vi "MCLB_AssertDisabledItems_Tests.vi"(11 "error in":errorcluster) -> (15 "error out":errorcluster)   [LabVIEW 2016, in "DronaTest.lvlib"]
uses:
  DronaTest.lvlib
  APIs/Stimulus/ControlValue/SetValueAuto.vi
  APIs/Assert/AssertControlValue/Controls/MC Listbox/AssertDisabledItems.vi
  <vilib>/addons/_JKI Toolkits/Caraya/classes/Assert/Assert Error.vi
  <vilib>/addons/_JKI Toolkits/Caraya/classes/Assert/Assert Equal Value_Variant.vi
  <vilib>/addons/_JKI Toolkits/Caraya/classes/Test/Test.lvclass
  Drona.lvlib
  <vilib>/SLL Toolkit/SLL Debug/SLL Debug.lvlib
  <vilib>/addons/_JKI Toolkits/Caraya/classes/Assert/Assert.lvclass
  APIs/Stimulus/ControlValue/ControlValue.lvlib
  APIs/Assert/AssertControlValue/Controls/MC Listbox/AssertMCListbox.lvlib
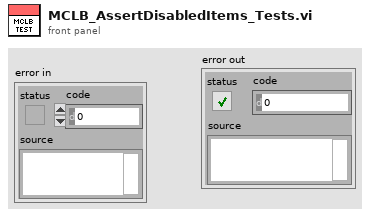
[diagram p1: front panel]
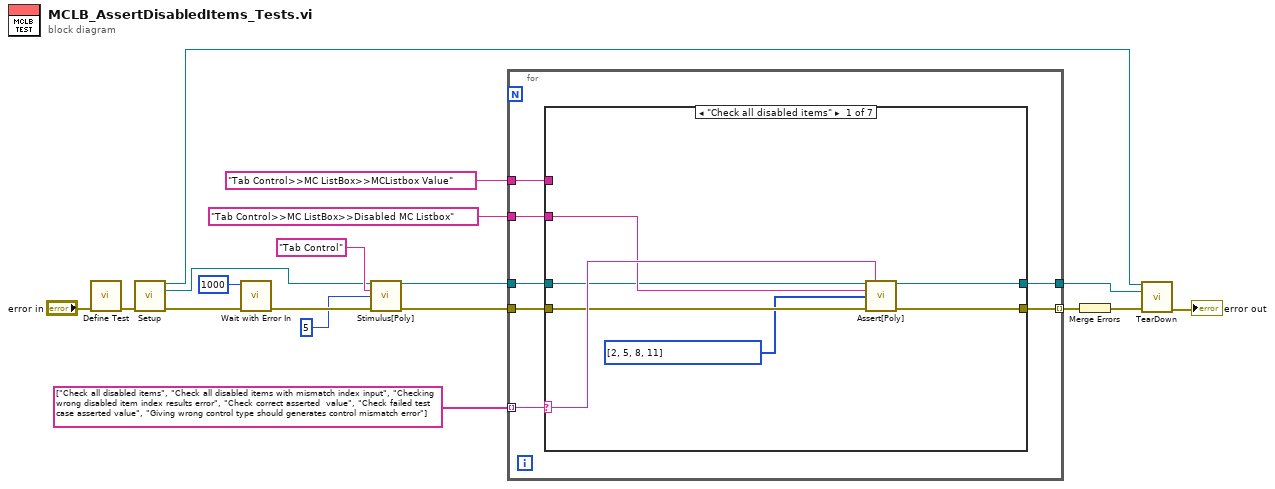
[diagram p0: block diagram]
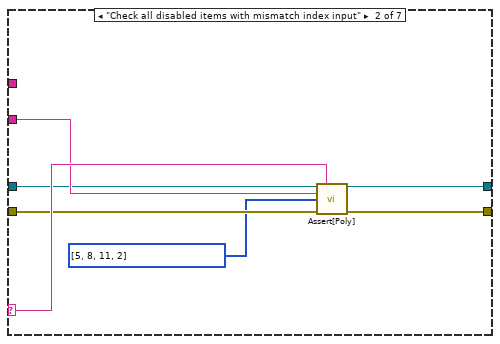
[diagram p2: hidden frame]
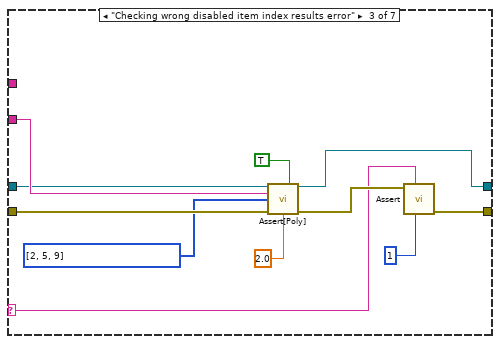
[diagram p3: hidden frame]
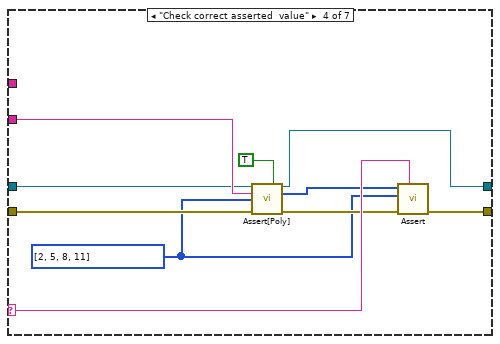
[diagram p4: hidden frame]
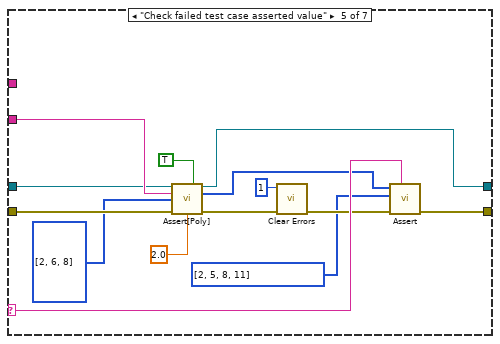
[diagram p5: hidden frame]
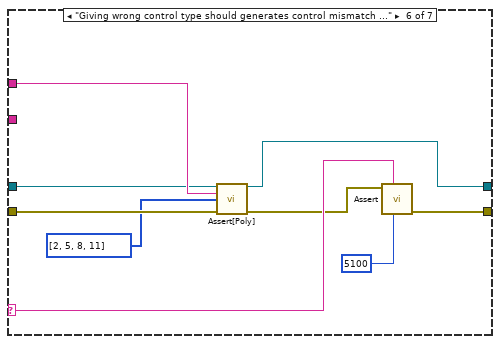
[diagram p6: hidden frame]
diagram:
  n1 = call <vilib>:"Define Test.vi"("error in (no error)"="error in") -> ("error out"=w7:errorcluster)  [unwired: 9 in, 1 out]
  n2 = call "Setup.vi"("error in (no error)"=w7) -> ("Application Ref"=w3:refnum<vi>, "VI out"=w5:refnum<vi>, "error out"=w6:errorcluster)  [unwired: 12 in]
  n3 = call <vilib>:"Wait with Error In.vi"("error in (no error)"=w6, "milliseconds to wait"=u32 1000) -> ("error out"=w16:errorcluster)  [unwired: 9 in]
  n4 = call-poly "Stimulus[Poly].vi"("VI Reference In"=w5, "Control Path"="Tab Control", "Value (Signaling)"=5, "error in"=w16) -> ("VI Reference Out"=w12:refnum<vi>, "error out"=w15:errorcluster)  [unwired: 10 in]
  n5 = for {
    tunnel: w12 -> [w24]
    tunnel: "Tab Control>>MC ListBox>>Disabled MC Listbox" ("Control Path") -> [w23]
    tunnel: "Tab Control>>MC ListBox>>MCListbox Value" ("Control Path") -> [w22]
    tunnel: string[] ["Check all disabled items", "Check all disabled items with mismatch index input", "Checking wrong disabled item index results error", "Check correct asserted  value", "Check failed test case asserted value", "Giving wrong control type should generates control mismatch error"] -> [w20] mode=indexing
    tunnel: [w19] -> w2
    tunnel: w15 -> [w25]
    tunnel: [w21] -> w8 mode=indexing
    n6 = case shown="\"Check all disabled items\"" w20 {
      selector: w20 -> [w30 w37 w43 w59 w73 w82 _]
      tunnel: w25 -> [w28 w35 w49 w55 w69 w77 w85]
      tunnel: w24 -> [w27 w34 w48 w54 w68 w76 w84]
      tunnel: w23 -> [w29 w36 w50 w58 w72 _ _]
      tunnel: w22 -> [_ _ _ _ _ w79 _]
      tunnel: [w32 w39 w45 w60 w74 w83 w85] -> w21
      tunnel: [w31 w38 w42 w57 w71 w78 w84] -> w19
      frame "Check all disabled items" {
        n7 = call-poly "Assert[Poly].vi"("VI Reference In"=w27, "Test Label"=w30, "Control Path"=w29, "Disabled Items"=i32[] [2, 5, 8, 11], "Error In"=w28) -> ("VI Reference Out"=w31:refnum<vi>, "Error Out"=w32:errorcluster)  [unwired: 8 in, 1 out]
      }
      frame "Check all disabled items with mismatch index input" {
        n8 = call-poly "Assert[Poly].vi"("VI Reference In"=w34, "Test Label"=w37, "Control Path"=w36, "Disabled Items"=i32[] [5, 8, 11, 2], "Error In"=w35) -> ("VI Reference Out"=w38:refnum<vi>, "Error Out"=w39:errorcluster)  [unwired: 8 in, 1 out]
      }
      frame "Checking wrong disabled item index results error" {
        n9 = call-poly "Assert[Poly].vi"("VI Reference In"=w48, "Assert Only? (F)"=TRUE, "Control Path"=w50, "Disabled Items"=i32[] [2, 5, 9], "Error In"=w49, "Timeout(5 sec)"=2.0) -> ("VI Reference Out"=w42:refnum<vi>, "Error Out"=w46:errorcluster)  [unwired: 7 in, 1 out]
        n10 = call-poly <vilib>:"Assert.vi"("error code (1)"=1, "Label"=w43, "Error?"=w46) -> ("error out"=w45:errorcluster)  [unwired: 7 in, 1 out]
      }
      frame "Check correct asserted  value" {
        w51 = i32[] [2, 5, 8, 11] ("Disabled Items")
        n11 = call-poly "Assert[Poly].vi"("VI Reference In"=w54, "Assert Only? (F)"=TRUE, "Control Path"=w58, "Disabled Items"=w51, "Error In"=w55) -> ("VI Reference Out"=w57:refnum<vi>, "Asserted Value"=w52:i32[], "Error Out"=w53:errorcluster)  [unwired: 8 in]
        n12 = call-poly <vilib>:"Assert.vi"("Label"=w59, "error in (no error)"=w53, "Y"=w51, "X"=w52) -> ("error out"=w60:errorcluster)  [unwired: 6 in, 1 out]
      }
      frame "Check failed test case asserted value" {
        n13 = call-poly "Assert[Poly].vi"("VI Reference In"=w68, "Assert Only? (F)"=TRUE, "Control Path"=w72, "Disabled Items"=i32[] [2, 6, 8], "Error In"=w69, "Timeout(5 sec)"=2.0) -> ("VI Reference Out"=w71:refnum<vi>, "Asserted Value"=w66:i32[], "Error Out"=w67:errorcluster)  [unwired: 7 in]
        n14 = call <vilib>:"Clear Errors.vi"("error in (no error)"=w67, "specific error code to clear (0: all)"=1) -> ("error out"=w65:errorcluster)  [unwired: 4 in, 1 out]
        n15 = call-poly <vilib>:"Assert.vi"("Label"=w73, "error in (no error)"=w65, "Y"=i32[] [2, 5, 8, 11] ("Disabled Items"), "X"=w66) -> ("error out"=w74:errorcluster)  [unwired: 6 in, 1 out]
      }
      frame "Giving wrong control type should generates control mismatch error" {
        n16 = call-poly "Assert[Poly].vi"("VI Reference In"=w76, "Control Path"=w79, "Disabled Items"=i32[] [2, 5, 8, 11], "Error In"=w77) -> ("VI Reference Out"=w78:refnum<vi>, "Error Out"=w80:errorcluster)  [unwired: 9 in, 1 out]
        n17 = call-poly <vilib>:"Assert.vi"("error code (1)"=5100, "Label"=w82, "Error?"=w80) -> ("error out"=w83:errorcluster)  [unwired: 7 in, 1 out]
      }
      frame Default {
      }
    }
  }
  n18 = Merge Errors(w8) -> (w4:errorcluster)
  n19 = call "TearDown.vi"("Application Ref"=w3, "VI in"=w2, "error in (no error)"=w4) -> ("error out"=→"error out":errorcluster)  [unwired: 12 in]
